vi "_043.vi"() -> ()   [LabVIEW 2024]
panel:
  out "Internet Connection Indicator :":bool
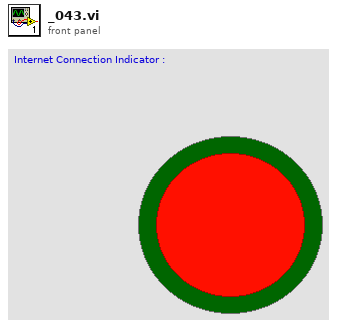
[diagram p1: front panel]
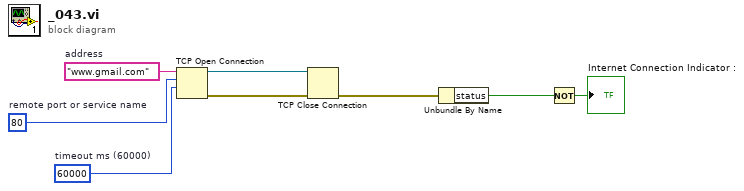
[diagram p0: block diagram]
diagram:
  w6 = 60000  # timeout ms (60000)
  w7 = u16 80  # remote port or service name
  w8 = "www.gmail.com"  # address
  n1 = TCP Open Connection(address=w8, remote port or service name=w7, timeout ms (60000)=w6) -> (connection ID=w5:refnum<k5>, error out=w4:errorcluster)  [unwired: 2 in]
  n2 = TCP Close Connection(connection ID=w5, error in (no error)=w4) -> (error out=w3:errorcluster)  [unwired: 1 in, 1 out]
  n3 = Unbundle By Name "Unbundle By Name"(w3) -> ("status"=w2:bool)
  n4 = Not(x=w2) -> (.not. x?=→"Internet Connection Indicator :":bool)
